vi "Rapid Read_NI.vi"(0 "NI Card":refnum<k15> caption="instrument handle", 3 "Channel":string="1", 5 "Motion Board ID":T1=1 min=1 max=32 step=1, 9 "rf points per line":i32, 11 "error in":errorcluster, 12 "timeout":dbl=1.0 format="%.2f", 14 "Pause?":bool) -> (1 "dig gain":dbl, 4 "Array":i8[][](array[numeric]), 6 "Reverse?":bool, 15 "error out":errorcluster)   [LabVIEW 2022 SP3]
uses:
  <instrlib>/niScope/Acquire/Fetch/niScope Multi Fetch Binary 8.vi
  <vilib>/DAQmx/write.llb/DAQmx Write (Digital Bool 1Line 1Point).vi
  Motion Controllers/-MotionRoutines/MotionGlobals.vi
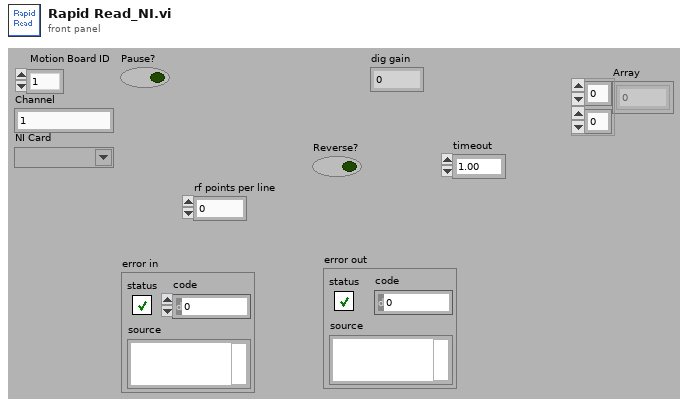
[diagram p1: front panel]
types:
  T1 = typedef "Board Id" = u8
  T2 = typedef "Var" = u8
  T3 = cluster{"actualSamples":i32, "absoluteInitialX":dbl, "relativeInitialX":dbl, "xIncrement":dbl, "offset":dbl, "gain":dbl, "reserved1":dbl, "reserved2":dbl}[]
  T4 = cluster{"actualSamples":i32, "absoluteInitialX":dbl, "relativeInitialX":dbl, "xIncrement":dbl, "offset":dbl, "gain":dbl, "reserved1":dbl, "reserved2":dbl}
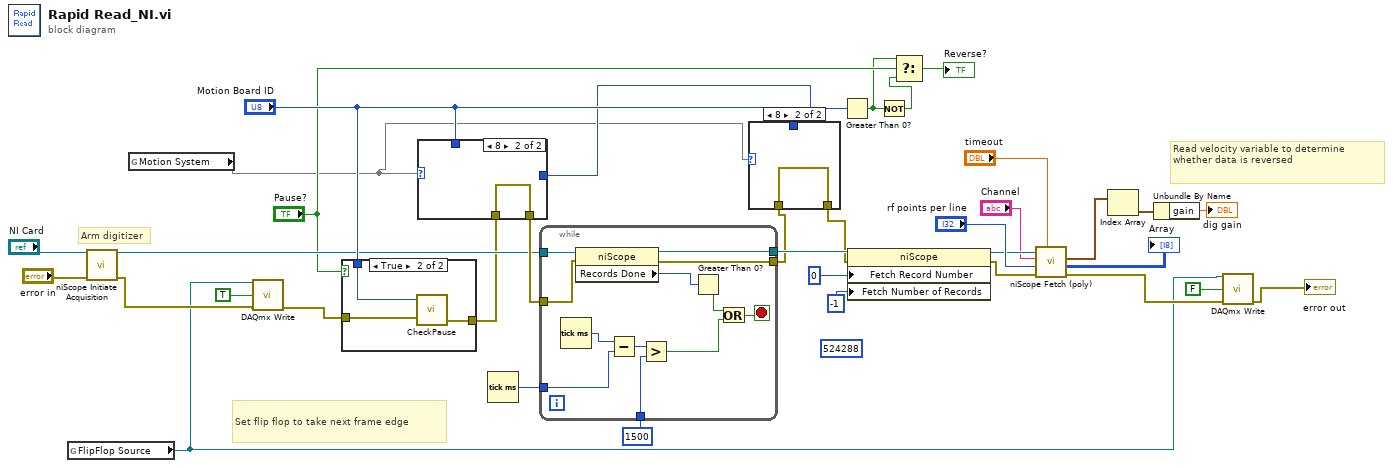
[diagram p0: block diagram]
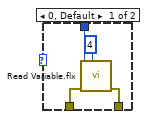
[diagram p2: hidden frame]
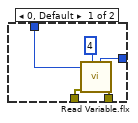
[diagram p3: hidden frame]
diagram:
  (unwired) 524288 ("Fetch:Data Transfer Block Size")
  # "Arm digitizer"
  # "Set flip flop to take next frame edge"
  # "Read velocity variable to determine whether data is reversed"
  n1 = global read "MotionGlobals.vi" "FlipFlop Source"() -> (w8:refnum<k21>)
  n2 = call <instrlib>:"niScope Initiate Acquisition.vi"("instrument handle"="NI Card", "error in"="error in") -> ("instrument handle out"=w7:refnum<k15>, "error out"=w13:errorcluster)  [unwired: 1 in, 11 out]
  n3 = global read "MotionGlobals.vi" "Motion System"() -> (w1)
  n4 = call-poly <vilib>:"DAQmx Write.vi"("task/channels in"=w8, "data"=TRUE ("stop (T)"), "error in"=w13) -> ("error out"=w12:errorcluster)  [unwired: 10 in, 2 out]
  n5 = case shown="True" "Pause?" {
    tunnel: w12 -> [w36 w39]
    tunnel: [w36 w38] -> w6
    tunnel: "Motion Board ID" -> [_ w37]
    frame False {
    }
    frame True {
      n6 = call "CheckPause.vi"("error in"=w39, "Motion Board ID"=w37) -> ("error out"=w38:errorcluster)  [unwired: 3 in]
    }
  }
  n7 = case shown="8" w1 {
    tunnel: [w43 w45] -> w17
    tunnel: "Motion Board ID" -> [w42 _]
    tunnel: [w41 _] -> w15
    tunnel: w6 -> [w40 w45]
    frame 0, Default {
      n8 = call <vilib>:"Read Variable.flx"("Var"=T2 4, "error in (no error)"=w40, "Board ID"=w42) -> ("error out"=w43:errorcluster, "Output"=w41:i32)  [unwired: 1 in, 4 out]
    }
    frame 8 {
    }
  }
  n9 = Tick Count (ms)() -> (millisecond timer value=w22:u32)
  n10 = while {
    tunnel: w7 -> [w57]
    tunnel: [w56] -> w23
    tunnel: w17 -> [w55]
    tunnel: [w54] -> w19
    tunnel: w22 -> [w52]
    tunnel: u32 1500 ("y") -> [w50]
    stop <- w48 stop-if-true
    n11 = Tick Count (ms)() -> (millisecond timer value=w53:u32)
    n12 = property class="niScope"(reference=w57, error in=w55) -> (reference out=w56:refnum<k15>, error out=w54:errorcluster, "Records Done"=w47:i32)
    n13 = Subtract(x=w53, y=w52) -> (x-y=w51:u32)
    n14 = Greater?(x=w51, y=w50) -> (0:w49:bool)
    n15 = Greater Than 0?(x=w47) -> (x > 0?=w46:bool)
    n16 = Or(x=w46, y=w49) -> (x .or. y?=w48:bool)
  }
  n17 = case shown="8" w1 {
    tunnel: w19 -> [w60 w62]
    tunnel: [w59 w62] -> w18
    tunnel: "Motion Board ID" -> [w58 _]
    frame 0, Default {
      n18 = call <vilib>:"Read Variable.flx"("Var"=T2 4, "error in (no error)"=w60, "Board ID"=w58) -> ("error out"=w59:errorcluster)  [unwired: 1 in, 5 out]
    }
    frame 8 {
    }
  }
  n19 = Greater Than 0?(x=w15) -> (x > 0?=w4:bool)
  n20 = property class="niScope"(reference=w23, error in=w18, "Fetch Record Number"=0, "Fetch Number of Records"=-1) -> (reference out=w29:refnum<k15>, error out=w28:errorcluster)
  n21 = Not(x=w4) -> (.not. x?=w3:bool)
  n22 = Select(t=w4, s="Pause?", f=w3) -> (s? t:f=→"Reverse?":bool)
  n23 = call-poly <instrlib>:"niScope Fetch (poly).vi"("timeout"="timeout", "error in"=w28, "numSamples"="rf points per line", "channels"="Channel", "instrument handle"=w29) -> ("error out"=w10:errorcluster, "wfm"=→"Array":i8[][], "wfm info"=w27:T3)  [unwired: 4 out]
  n24 = Index Array(array=w27) -> (element=w26:T4)  [unwired: 1 in]
  n25 = Unbundle By Name(w26) -> ("gain"=→"dig gain":dbl)
  n26 = call-poly <vilib>:"DAQmx Write.vi"("task/channels in"=w8, "data"=FALSE ("stop (T)"), "error in"=w10) -> ("error out"=→"error out":errorcluster)  [unwired: 10 in, 2 out]
